vi "emi_Time Diff Monitoring w Array.vi"(5 "Timing Info in":T1, 9 "error in (no error)":errorcluster) -> (6 "Timing Info out":cluster{"Differences":u32[], "Time":u32}, 8 "Differences":u32[](array[numeric]), 10 "error out":errorcluster)   [LabVIEW 2010]
doc: "Use this to se the number of ms an action takes. They need be chained together for full effect.\n\nTiming infor must be connected between all. On the last one use \"Time Differences out\" to see a list of differences."
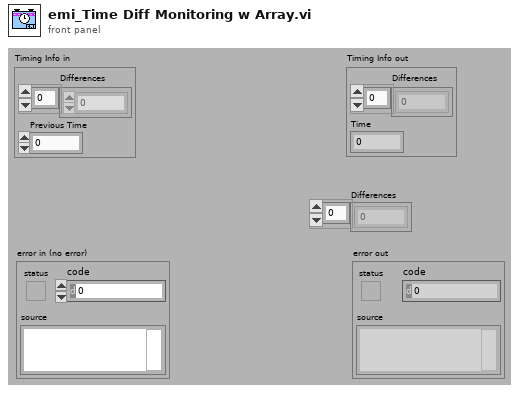
[diagram p1: front panel]
types:
  T1 = cluster{"Differences":u32[], "Previous Time":u32}
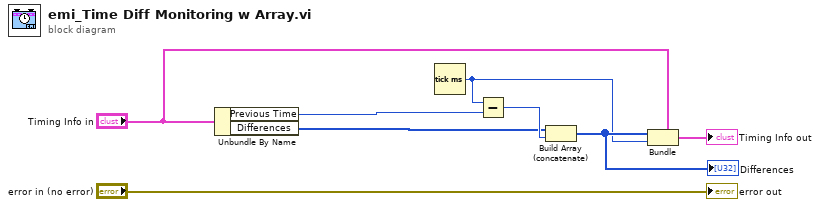
[diagram p0: block diagram]
diagram:
  n1 = Unbundle By Name("Timing Info in") -> ("Previous Time"=w6:u32, "Differences"=w5:u32[])
  n2 = Tick Count (ms)() -> (millisecond timer value=w2:u32)
  n3 = Subtract(x=w2, y=w6) -> (x-y=w7:u32)
  n4 = Build Array (concatenate)(w5, w7) -> (w3:u32[])
  "Differences" <- w3
  n5 = Bundle(cluster="Timing Info in", "Differences"=w3, "Previous Time"=w2) -> (→"Timing Info out":T1)
  "error out" <- "error in (no error)"
